vi "Get Camera Object.vi"() -> (0 "error out":errorcluster, 3 "Camera out":refnum<class "Camera.lvclass">)   [LabVIEW 2016, in "Camera.lvclass"]
uses:
  Camera.lvclass
  Edmund Optics/Edmund Optics.lvclass
  C:/Users/HEP Gantry/Documents/Assembly/V4/Classes/Controller/Camera/Camera.lvclass
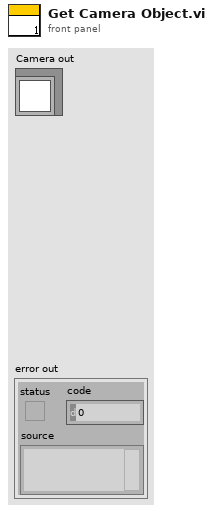
[diagram p1: front panel]
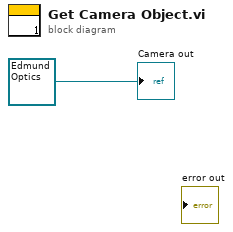
[diagram p0: block diagram]
diagram:
  "Camera out" <- refnum<class "Edmund Optics.lvclass"> refnum ("Edmund Optics.lvclass")
